vi "Format CSV.vi"(8 "error in (no error)":errorcluster, 9 "delimiter":string=",", 10 "CSV File Input":path, 11 "Original CSV Format":enum16{"Format A", "Format B"}(ring)) -> (0 "error out":errorcluster, 1 "Parcel Length":i32[](array[numeric]), 2 "All Terminal Data":T1(array[cluster]))   [LabVIEW 2017] (continued)
"38:45.8", "38:45.9", "38:45.9", "38:45.9", "38:46.0", "38:46.0", "38:46.0", "38:46.1", "38:46.1", "38:46.1", "38:46.2", "38:46.2", "38:46.2", "38:46.3", "38:46.3", "38:46.3", "38:46.4", "38:46.4", "38:46.4", "38:46.5", "38:46.5", "38:46.5", "38:46.6", "38:46.6", "38:46.6", "38:46.7", "38:46.7", "38:46.7", "38:46.8", "38:46.8", "38:46.8", "38:46.9", "38:46.9", "38:46.9", "38:47.0", "38:47.0", "38:47.0", "38:47.1", "38:47.1", "38:47.1", "38:47.2", "38:47.2", "38:47.2", "38:47.3", "38:47.3", "38:47.3", "38:47.4", "38:47.4", "38:47.4", "38:47.5", "38:47.5", "38:47.5", "38:47.6", "38:47.6", "38:47.6", "38:47.7", "38:47.7", "38:47.7", "38:47.8", "38:47.8", "38:47.8", "38:47.9", "38:47.9", "38:47.9", "38:48.0", "38:48.0", "38:48.0", "38:48.1", "38:48.1", "38:48.1", "38:48.2", "38:48.2", "38:48.2", "38:48.3", "38:48.3", "38:48.3", "38:48.4", "38:48.4", "38:48.4", "38:48.5", "38:48.5", "38:48.5", "38:48.6", "38:48.6", "38:48.6", "38:48.7", "38:48.7", "38:48.7", "38:48.8", "38:48.8", "38:48.8", "38:48.9", "38:48.9", "38:48.9", "38:49.0", "38:49.0", "38:49.0", "38:49.1", "38:49.1", "38:49.1", "38:49.2", "38:49.2", "38:49.2", "38:49.3", "38:49.3", "38:49.3", "38:49.4", "38:49.4", "38:49.4", "38:49.5", "38:49.5", "38:49.5", "38:49.6", "38:49.6", "38:49.6", "38:49.7", "38:49.7", "38:49.7", "38:49.8", "38:49.8", "38:49.8", "38:49.9", "38:49.9", "38:49.9", "38:50.0", "38:50.0", "38:50.0", "38:50.1", "38:50.1", "38:50.1", "38:50.2", "38:50.2", "38:50.2", "38:50.3", "38:50.3", "38:50.3", "38:50.4", "38:50.4", "38:50.4", "38:50.5", "38:50.5", "38:50.5", "38:50.6", "38:50.6", "38:50.6", "38:50.7", "38:50.7", "38:50.7", "38:50.8", "38:50.8", "38:50.8", "38:50.9", "38:50.9", "38:50.9", "38:51.0", "38:51.0", "38:51.0", "38:51.1", "38:51.1", "38:51.1", "38:51.2", "38:51.2", "38:51.2", "38:51.3", "38:51.3", "38:51.3", "38:51.4", "38:51.4", "38:51.4", "38:51.5", "38:51.5", "38:51.5", "38:51.6", "38:51.6", "38:51.6", "38:51.7", "38:51.7", "38:51.7", "38:51.8", "38:51.8", "38:51.8", "38:51.9", "38:51.9", "38:51.9", "38:52.0", "38:52.0", "38:52.0", "38:52.1", "38:52.1", "38:52.1", "38:52.2", "38:52.2", "38:52.2", "38:52.3", "38:52.3", "38:52.3", "38:52.4", "38:52.4", "38:52.4", "38:52.5", "38:52.5", "38:52.5", "38:52.6", "38:52.6", "38:52.6", "38:52.7", "38:52.7", "38:52.7", "38:52.8", "38:52.8", "38:52.8", "38:52.9", "38:52.9", "38:52.9", "38:53.0", "38:53.0", "38:53.0", "38:53.1", "38:53.1", "38:53.1", "38:53.2", "38:53.2", "38:53.2", "38:53.3", "38:53.3", "38:53.3", "38:53.4", "38:53.4", "38:53.4", "38:53.5", "38:53.5", "38:53.5", "38:53.6", "38:53.6", "38:53.6", "38:53.7", "38:53.7", "38:53.7", "38:53.8", "38:53.8", "38:53.8", "38:53.9", "38:53.9", "38:53.9", "38:54.0", "38:54.0", "38:54.0", "38:54.1", "38:54.1", "38:54.1", "38:54.2", "38:54.2", "38:54.2", "38:54.3", "38:54.3", "38:54.3", "38:54.4", "38:54.4", "38:54.4", "38:54.5", "38:54.5", "38:54.5", "38:54.6", "38:54.6", "38:54.6", "38:54.7", "38:54.7", "38:54.7", "38:54.8", "38:54.8", "38:54.8", "38:54.9", "38:54.9", "38:54.9", "38:55.0", "38:55.0", "38:55.0", "38:55.1", "38:55.1", "38:55.1", "38:55.2", "38:55.2", "38:55.2", "38:55.3", "38:55.3", "38:55.3", "38:55.4", "38:55.4", "38:55.4", "38:55.5", "38:55.5", "38:55.5", "38:55.6", "38:55.6", "38:55.6", "38:55.7", "38:55.7", "38:55.7", "38:55.8", "38:55.8", "38:55.8", "38:55.9", "38:55.9", "38:55.9", "38:56.0", "38:56.0", "38:56.0", "38:56.1", "38:56.1", "38:56.1", "38:56.2", "38:56.2", "38:56.2", "38:56.3", "38:56.3", "38:56.3", "38:56.4", "38:56.4", "38:56.4", "38:56.5", "38:56.5", "38:56.5", "38:56.6", "38:56.6", "38:56.6", "38:56.7", "38:56.7", "38:56.7", "38:56.8", "38:56.8", "38:56.8", "38:56.9", "38:56.9", "38:56.9", "38:57.0", "38:57.0", "38:57.0", "38:57.1", "38:57.1", "38:57.1", "38:57.2", "38:57.2", "38:57.2", "38:57.3", "38:57.3", "38:57.3", "38:57.4", "38:57.4", "38:57.4", "38:57.5", "38:57.5", "38:57.5", "38:57.6", "38:57.6", "38:57.6", "38:57.7", "38:57.7", "38:57.7", "38:57.8", "38:57.8", "38:57.8", "38:57.9", "38:57.9", "38:57.9", "38:58.0", "38:58.0", "38:58.0", "38:58.1", "38:58.1", "38:58.1", "38:58.2", "38:58.2", "38:58.2", "38:58.3", "38:58.3", "38:58.3", "38:58.4", "38:58.4", "38:58.4", "38:58.5", "38:58.5", "38:58.5", "38:58.6", "38:58.6", "38:58.6", "38:58.7", "38:58.7", "38:58.7", "38:58.8", "38:58.8", "38:58.8", "38:58.9", "38:58.9", "38:58.9", "38:59.0", "38:59.0", "38:59.0", "38:59.1", "38:59.1", "38:59.1", "38:59.2", "38:59.2", "38:59.2", "38:59.3", "38:59.3", "38:59.3", "38:59.4", "38:59.4", "38:59.4", "38:59.5", "38:59.5", "38:59.5", "38:59.6", "38:59.6", "38:59.6", "38:59.7", "38:59.7", "38:59.7", "38:59.8", "38:59.8", "38:59.8", "38:59.9", "38:59.9", "38:59.9", "39:00.0", "39:00.0", "39:00.0", "39:00.1", "39:00.1", "39:00.1", "39:00.2", "39:00.2", "39:00.2", "39:00.3", "39:00.3", "39:00.3", "39:00.4", "39:00.4", "39:00.4", "39:00.5", "39:00.5", "39:00.5", "39:00.6", "39:00.6", "39:00.6", "39:00.7", "39:00.7", "39:00.7", "39:00.8", "39:00.8", "39:00.8", "39:00.9", "39:00.9", "39:00.9", "39:01.0", "39:01.0", "39:01.0", "39:01.1", "39:01.1", "39:01.1", "39:01.2", "39:01.2", "39:01.2", "39:01.3", "39:01.3", "39:01.3", "39:01.4", "39:01.4", "39:01.4", "39:01.5", "39:01.5", "39:01.5", "39:01.6", "39:01.6", "39:01.6", "39:01.7", "39:01.7", "39:01.7", "39:01.8", "39:01.8", "39:01.8", "39:01.9", "39:01.9", "39:01.9", "39:02.0", "39:02.0", "39:02.0", "39:02.1", "39:02.1", "39:02.1", "39:02.2", "39:02.2", "39:02.2", "39:02.3", "39:02.3", "39:02.3", "39:02.4", "39:02.4", "39:02.4", "39:02.5", "39:02.5", "39:02.5", "39:02.6", "39:02.6", "39:02.6", "39:02.7", "39:02.7", "39:02.7", "39:02.8", "39:02.8", "39:02.8", "39:02.9", "39:02.9", "39:02.9", "39:03.0", "39:03.0", "39:03.0", "39:03.1", "39:03.1", "39:03.1", "39:03.2", "39:03.2", "39:03.2", "39:03.3", "39:03.3", "39:03.3", "39:03.4", "39:03.4", "39:03.4", "39:03.5", "39:03.5", "39:03.5", "39:03.6", "39:03.6", "39:03.6", "39:03.7", "39:03.7", "39:03.7", "39:03.8", "39:03.8", "39:03.8", "39:03.9", "39:03.9", "39:03.9", "39:04.0", "39:04.0", "39:04.0", "39:04.1", "39:04.1", "39:04.1", "39:04.2", "39:04.2", "39:04.2", "39:04.3", "39:04.3", "39:04.3", "39:04.4", "39:04.4", "39:04.4", "39:04.5", "39:04.5", "39:04.5", "39:04.6", "39:04.6", "39:04.6", "39:04.7", "39:04.7", "39:04.7", "39:04.8", "39:04.8", "39:04.8", "39:04.9", "39:04.9", "39:04.9", "39:05.0", "39:05.0", "39:05.0", "39:05.1", "39:05.1", "39:05.1", "39:05.2", "39:05.2", "39:05.2", "39:05.3", "39:05.3", "39:05.3", "39:05.4", "39:05.4", "39:05.4", "39:05.5", "39:05.5", "39:05.5", "39:05.6", "39:05.6", "39:05.6", "39:05.7", "39:05.7", "39:05.7", "39:05.8", "39:05.8", "39:05.8", "39:05.9", "39:05.9", "39:05.9", "39:06.0", "39:06.0", "39:06.0", "39:06.1", "39:06.1", "39:06.1", "39:06.2", "39:06.2", "39:06.2", "39:06.3", "39:06.3", "39:06.3", "39:06.4", "39:06.4", "39:06.4", "39:06.5", "39:06.5", "39:06.5", "39:06.6", "39:06.6", "39:06.6", "39:06.7", "39:06.7", "39:06.7", "39:06.8", "39:06.8", "39:06.8", "39:06.9", "39:06.9", "39:06.9", "39:07.0", "39:07.0", "39:07.0", "39:07.1", "39:07.1", "39:07.1", "39:07.2", "39:07.2", "39:07.2", "39:07.3", "39:07.3", "39:07.3", "39:07.4", "39:07.4", "39:07.4", "39:07.5", "39:07.5", "39:07.5", "39:07.6", "39:07.6", "39:07.6", "39:07.7", "39:07.7", "39:07.7", "39:07.8", "39:07.8", "39:07.8", "39:07.9", "39:07.9", "39:07.9", "39:08.0", "39:08.0", "39:08.0", "39:08.1", "39:08.1", "39:08.1", "39:08.2", "39:08.2", "39:08.2", "39:08.3", "39:08.3", "39:08.3", "39:08.4", "39:08.4", "39:08.4", "39:08.5", "39:08.5", "39:08.5", "39:08.6", "39:08.6", "39:08.6", "39:08.7", "39:08.7", "39:08.7", "39:08.8", "39:08.8", "39:08.8", "39:08.9", "39:08.9", "39:08.9", "39:09.0", "39:09.0", "39:09.0", "39:09.1", "39:09.1", "39:09.1", "39:09.2", "39:09.2", "39:09.2", "39:09.3", "39:09.3", "39:09.3", "39:09.4", "39:09.4", "39:09.4", "39:09.5", "39:09.5", "39:09.5", "39:09.6", "39:09.6", "39:09.6", "39:09.7", "39:09.7", "39:09.7", "39:09.8", "39:09.8", "39:09.8", "39:09.9", "39:09.9", "39:09.9", "39:10.0", "39:10.0", "39:10.0", "39:10.1", "39:10.1", "39:10.1", "39:10.2", "39:10.2", "39:10.2", "39:10.3", "39:10.3", "39:10.3", "39:10.4", "39:10.4", "39:10.4", "39:10.5", "39:10.5", "39:10.5", "39:10.6", "39:10.6", "39:10.6", "39:10.7", "39:10.7", "39:10.7", "39:10.8", "39:10.8", "39:10.8", "39:10.9", "39:10.9", "39:10.9", "39:11.0", "39:11.0", "39:11.0", "39:11.1", "39:11.1", "39:11.1", "39:11.2", "39:11.2", "39:11.2", "39:11.3", "39:11.3", "39:11.3", "39:11.4", "39:11.4", "39:11.4", "39:11.5", "39:11.5", "39:11.5", "39:11.6", "39:11.6", "39:11.6", "39:11.7", "39:11.7", "39:11.7", "39:11.8", "39:11.8", "39:11.8", "39:11.9", "39:11.9", "39:11.9", "39:12.0", "39:12.0", "39:12.0", "39:12.1", "39:12.1", "39:12.1", "39:12.2", "39:12.2", "39:12.2", "39:12.3", "39:12.3", "39:12.3", "39:12.4", "39:12.4", "39:12.4", "39:12.5", "39:12.5", "39:12.5", "39:12.6", "39:12.6", "39:12.6", "39:12.7", "39:12.7", "39:12.7", "39:12.8", "39:12.8", "39:12.8", "39:12.9", "39:12.9", "39:12.9", "39:13.0", "39:13.0", "39:13.0", "39:13.1", "39:13.1", "39:13.1", "39:13.2", "39:13.2", "39:13.2", "39:13.3", "39:13.3", "39:13.3", "39:13.4", "39:13.4", "39:13.4", "39:13.5", "39:13.5", "39:13.5", "39:13.6", "39:13.6", "39:13.6", "39:13.7", "39:13.7", "39:13.7", "39:13.8", "39:13.8", "39:13.8", "39:13.9", "39:13.9", "39:13.9", "39:14.0", "39:14.0", "39:14.0", "39:14.1", "39:14.1", "39:14.1", "39:14.2", "39:14.2", "39:14.2", "39:14.3", "39:14.3", "39:14.3", "39:14.4", "39:14.4", "39:14.4", "39:14.5", "39:14.5", "39:14.5", "39:14.6", "39:14.6", "39:14.6", "39:14.7", "39:14.7", "39:14.7", "39:14.8", "39:14.8", "39:14.8", "39:14.9", "39:14.9", "39:14.9", "39:15.0", "39:15.0", "39:15.0", "39:15.1", "39:15.1", "39:15.1", "39:15.2", "39:15.2", "39:15.2", "39:15.3", "39:15.3", "39:15.3", "39:15.4", "39:15.4", "39:15.4", "39:15.5", "39:15.5", "39:15.5", "39:15.6", "39:15.6", "39:15.6", "39:15.7", "39:15.7", "39:15.7", "39:15.8", "39:15.8", "39:15.8", "39:15.9", "39:15.9", "39:15.9", "39:16.0", "39:16.0", "39:16.0", "39:16.1", "39:16.1", "39:16.1", "39:16.2", "39:16.2", "39:16.2", "39:16.3", "39:16.3", "39:16.3", "39:16.4", "39:16.4", "39:16.4", "39:16.5", "39:16.5", "39:16.5", "39:16.6", "39:16.6", "39:16.6", "39:16.7", "39:16.7", "39:16.7", "39:16.8", "39:16.8", "39:16.8", "39:16.9", "39:16.9", "39:16.9", "39:17.0", "39:17.0", "39:17.0", "39:17.1", "39:17.1", "39:17.1", "39:17.2", "39:17.2", "39:17.2", "39:17.3", "39:17.3", "39:17.3", "39:17.4", "39:17.4", "39:17.4", "39:17.5", "39:17.5", "39:17.5", "39:17.6", "39:17.6", "39:17.6", "39:17.7", "39:17.7", "39:17.7", "39:17.8", "39:17.8", "39:17.8", "39:17.9", "39:17.9", "39:17.9", "39:18.0", "39:18.0", "39:18.0", "39:18.1", "39:18.1", "39:18.1", "39:18.2", "39:18.2", "39:18.2", "39:18.3", "39:18.3", "39:18.3", "39:18.4", "39:18.4", "39:18.4", "39:18.5", "39:18.5", "39:18.5", "39:18.6", "39:18.6", "39:18.6", "39:18.7", "39:18.7", "39:18.7", "39:18.8", "39:18.8", "39:18.8", "39:18.9", "39:18.9", "39:18.9", "39:19.0", "39:19.0", "39:19.0", "39:19.1", "39:19.1", "39:19.1", "39:19.2", "39:19.2", "39:19.2", "39:19.3", "39:19.3", "39:19.3", "39:19.4", "39:19.4", "39:19.4", "39:19.5", "39:19.5", "39:19.5", "39:19.6", "39:19.6", "39:19.6", "39:19.7", "39:19.7", "39:19.7", "39:19.8", "39:19.8", "39:19.8", "39:19.9", "39:19.9", "39:19.9", "39:20.0", "39:20.0", "39:20.0", "39:20.1", "39:20.1", "39:20.1", "39:20.2", "39:20.2", "39:20.2", "39:20.3", "39:20.3", "39:20.3", "39:20.4", "39:20.4", "39:20.4", "39:20.5", "39:20.5", "39:20.5", "39:20.6", "39:20.6", "39:20.6", "39:20.7", "39:20.7", "39:20.7", "39:20.8", "39:20.8", "39:20.8", "39:20.9", "39:20.9", "39:20.9", "39:21.0", "39:21.0", "39:21.0", "39:21.1", "39:21.1", "39:21.1", "39:21.2", "39:21.2", "39:21.2", "39:21.3", "39:21.3", "39:21.3", "39:21.4", "39:21.4", "39:21.4", "39:21.5", "39:21.5", "39:21.5", "39:21.6", "39:21.6", "39:21.6", "39:21.7", "39:21.7", "39:21.7", "39:21.8", "39:21.8", "39:21.8", "39:21.9", "39:21.9", "39:21.9", "39:22.0", "39:22.0", "39:22.0", "39:22.1", "39:22.1", "39:22.1", "39:22.2", "39:22.2", "39:22.2", "39:22.3", "39:22.3", "39:22.3", "39:22.4", "39:22.4", "39:22.4", "39:22.5", "39:22.5", "39:22.5", "39:22.6", "39:22.6", "39:22.6", "39:22.7", "39:22.7", "39:22.7", "39:22.8", "39:22.8", "39:22.8", "39:22.9", "39:22.9", "39:22.9", "39:23.0", "39:23.0", "39:23.0", "39:23.1", "39:23.1", "39:23.1", "39:23.2", "39:23.2", "39:23.2", "39:23.3", "39:23.3", "39:23.3", "39:23.4", "39:23.4", "39:23.4", "39:23.5", "39:23.5", "39:23.5", "39:23.6", "39:23.6", "39:23.6", "39:23.7", "39:23.7", "39:23.7", "39:23.8", "39:23.8", "39:23.8", "39:23.9", "39:23.9", "39:23.9", "39:24.0", "39:24.0", "39:24.0", "39:24.1", "39:24.1", "39:24.1", "39:24.2", "39:24.2", "39:24.2", "39:24.3", "39:24.3", "39:24.3", "39:24.4", "39:24.4", "39:24.4", "39:24.5", "39:24.5", "39:24.5", "39:24.6", "39:24.6", "39:24.6", "39:24.7", "39:24.7", "39:24.7", "39:24.8", "39:24.8", "39:24.8", "39:24.9", "39:24.9", "39:24.9", "39:25.0", "39:25.0", "39:25.0", "39:25.1", "39:25.1", "39:25.1", "39:25.2", "39:25.2", "39:25.2", "39:25.3", "39:25.3", "39:25.3", "39:25.4", "39:25.4", "39:25.4", "39:25.5", "39:25.5", "39:25.5", "39:25.6", "39:25.6", "39:25.6", "39:25.7", "39:25.7", "39:25.7", "39:25.8", "39:25.8", "39:25.8", "39:25.9", "39:25.9", "39:25.9", "39:26.0", "39:26.0", "39:26.0", "39:26.1", "39:26.1", "39:26.1", "39:26.2", "39:26.2", "39:26.2", "39:26.3", "39:26.3", "39:26.3", "39:26.4", "39:26.4", "39:26.4", "39:26.5", "39:26.5", "39:26.5", "39:26.6", "39:26.6", "39:26.6", "39:26.7", "39:26.7", "39:26.7", "39:26.8", "39:26.8", "39:26.8", "39:26.9", "39:26.9", "39:26.9", "39:27.0", "39:27.0", "39:27.0", "39:27.1", "39:27.1", "39:27.1", "39:27.2", "39:27.2", "39:27.2", "39:27.3", "39:27.3", "39:27.3", "39:27.4", "39:27.4", "39:27.4", "39:27.5", "39:27.5", "39:27.5", "39:27.6", "39:27.6", "39:27.6", "39:27.7", "39:27.7", "39:27.7", "39:27.8", "39:27.8", "39:27.8", "39:27.9", "39:27.9", "39:27.9", "39:28.0", "39:28.0", "39:28.0", "39:28.1", "39:28.1", "39:28.1", "39:28.2", "39:28.2", "39:28.2", "39:28.3", "39:28.3", "39:28.3", "39:28.4", "39:28.4", "39:28.4", "39:28.5", "39:28.5", "39:28.5", "39:28.6", "39:28.6", "39:28.6", "39:28.7", "39:28.7", "39:28.7", "39:28.8", "39:28.8", "39:28.8", "39:28.9", "39:28.9", "39:28.9", "39:29.0", "39:29.0", "39:29.0", "39:29.1", "39:29.1", "39:29.1", "39:29.2", "39:29.2", "39:29.2", "39:29.3", "39:29.3", "39:29.3", "39:29.4", "39:29.4", "39:29.4", "39:29.5", "39:29.5", "39:29.5", "39:29.6", "39:29.6", "39:29.6", "39:29.7", "39:29.7", "39:29.7", "39:29.8", "39:29.8", "39:29.8", "39:29.9", "39:29.9", "39:29.9", "39:30.0", "39:30.0", "39:30.0", "39:30.1", "39:30.1", "39:30.1", "39:30.2", "39:30.2", "39:30.2", "39:30.3", "39:30.3", "39:30.3", "39:30.4", "39:30.4", "39:30.4", "39:30.5", "39:30.5", "39:30.5", "39:30.6", "39:30.6", "39:30.6", "39:30.7", "39:30.7", "39:30.7", "39:30.8", "39:30.8", "39:30.8", "39:30.9", "39:30.9", "39:30.9", "39:31.0", "39:31.0", "39:31.0", "39:31.1", "39:31.1", "39:31.1", "39:31.2", "39:31.2", "39:31.2", "39:31.3", "39:31.3", "39:31.3", "39:31.4", "39:31.4", "39:31.4", "39:31.5", "39:31.5", "39:31.5", "39:31.6", "39:31.6", "39:31.6", "39:31.7", "39:31.7", "39:31.7", "39:31.8", "39:31.8", "39:31.8", "39:31.9", "39:31.9", "39:31.9", "39:32.0", "39:32.0", "39:32.0", "39:32.1", "39:32.1", "39:32.1", "39:32.2", "39:32.2", "39:32.2", "39:32.3", "39:32.3", "39:32.3", "39:32.4", "39:32.4", "39:32.4", "39:32.5", "39:32.5", "39:32.5", "39:32.6", "39:32.6", "39:32.6", "39:32.7", "39:32.7", "39:32.7", "39:32.8", "39:32.8", "39:32.8", "39:32.9", "39:32.9", "39:32.9", "39:33.0", "39:33.0", "39:33.0", "39:33.1", "39:33.1", "39:33.1", "39:33.2", "39:33.2", "39:33.2", "39:33.3", "39:33.3", "39:33.3", "39:33.4", "39:33.4", "39:33.4", "39:33.5", "39:33.5", "39:33.5", "39:33.6", "39:33.6", "39:33.6", "39:33.7", "39:33.7", "39:33.7", "39:33.8", "39:33.8", "39:33.8", "39:33.9", "39:33.9", "39:33.9", "39:34.0", "39:34.0", "39:34.0", "39:34.1", "39:34.1", "39:34.1", "39:34.2", "39:34.2", "39:34.2", "39:34.3", "39:34.3", "39:34.3", "39:34.4", "39:34.4", "39:34.4", "39:34.5", "39:34.5", "39:34.5", "39:34.6", "39:34.6", "39:34.6", "39:34.7", "39:34.7", "39:34.7", "39:34.8", "39:34.8", "39:34.8", "39:34.9", "39:34.9", "39:34.9", "39:35.0", "39:35.0", "39:35.0", "39:35.1", "39:35.1", "39:35.1", "39:35.2", "39:35.2", "39:35.2", "39:35.3", "39:35.3", "39:35.3", "39:35.4", "39:35.4", "39:35.4", "39:35.5", "39:35.5", "39:35.5", "39:35.6", "39:35.6", "39:35.6", "39:35.7", "39:35.7", "39:35.7", "39:35.8", "39:35.8", "39:35.8", "39:35.9", "39:35.9", "39:35.9", "39:36.0", "39:36.0", "39:36.0", "39:36.1", "39:36.1", "39:36.1", "39:36.2", "39:36.2", "39:36.2", "39:36.3", "39:36.3", "39:36.3", "39:36.4", "39:36.4", "39:36.4", "39:36.5", "39:36.5", "39:36.5", "39:36.6", "39:36.6", "39:36.6", "39:36.7", "39:36.7", "39:36.7", "39:36.8", "39:36.8", "39:36.8", "39:36.9", "39:36.9", "39:36.9", "39:37.0", "39:37.0", "39:37.0", "39:37.1", "39:37.1", "39:37.1", "39:37.2", "39:37.2", "39:37.2", "39:37.3", "39:37.3", "39:37.3", "39:37.4", "39:37.4", "39:37.4", "39:37.5", "39:37.5", "39:37.5", "39:37.6", "39:37.6", "39:37.6", "39:37.7", "39:37.7", "39:37.7", "39:37.8", "39:37.8", "39:37.8", "39:37.9", "39:37.9", "39:37.9", "39:38.0", "39:38.0", "39:38.0", "39:38.1", "39:38.1", "39:38.1", "39:38.2", "39:38.2", "39:38.2", "39:38.3", "39:38.3", "39:38.3", "39:38.4", "39:38.4", "39:38.4", "39:38.5", "39:38.5", "39:38.5", "39:38.6", "39:38.6", "39:38.6", "39:38.7", "39:38.7", "39:38.7", "39:38.8", "39:38.8", "39:38.8", "39:38.9", "39:38.9", "39:38.9", "39:39.0", "39:39.0", "39:39.0", "39:39.1", "39:39.1", "39:39.1", "39:39.2", "39:39.2", "39:39.2", "39:39.3", "39:39.3", "39:39.3", "39:39.4", "39:39.4", "39:39.4", "39:39.5", "39:39.5", "39:39.5", "39:39.6", "39:39.6", "39:39.6", "39:39.7", "39:39.7", "39:39.7", "39:39.8", "39:39.8", "39:39.8", "39:39.9", "39:39.9", "39:39.9", "39:40.0", "39:40.0", "39:40.0", "39:40.1", "39:40.1", "39:40.1", "39:40.2", "39:40.2", "39:40.2", "39:40.3", "39:40.3", "39:40.3", "39:40.4", "39:40.4", "39:40.4", "39:40.5", "39:40.5", "39:40.5", "39:40.6", "39:40.6", "39:40.6", "39:40.7", "39:40.7", "39:40.7", "39:40.8", "39:40.8", "39:40.8", "39:40.9", "39:40.9", "39:40.9", "39:41.0", "39:41.0", "39:41.0", "39:41.1", "39:41.1", "39:41.1", "39:41.2", "39:41.2", "39:41.2", "39:41.3", "39:41.3", "39:41.3", "39:41.4", "39:41.4", "39:41.4", "39:41.5", "39:41.5", "39:41.5", "39:41.6", "39:41.6", "39:41.6", "39:41.7", "39:41.7", "39:41.7", "39:41.8", "39:41.8", "39:41.8", "39:41.9", "39:41.9", "39:41.9", "39:42.0", "39:42.0", "39:42.0", "39:42.1", "39:42.1", "39:42.1", "39:42.2", "39:42.2", "39:42.2", "39:42.3", "39:42.3", "39:42.3", "39:42.4", "39:42.4", "39:42.4", "39:42.5", "39:42.5", "39:42.5", "39:42.6", "39:42.6", "39:42.6", "39:42.7", "39:42.7", "39:42.7", "39:42.8", "39:42.8", "39:42.8", "39:42.9", "39:42.9", "39:42.9", "39:43.0", "39:43.0", "39:43.0", "39:43.1", "39:43.1", "39:43.1", "39:43.2", "39:43.2", "39:43.2", "39:43.3", "39:43.3", "39:43.3", "39:43.4", "39:43.4", "39:43.4", "39:43.5", "39:43.5", "39:43.5", "39:43.6", "39:43.6", "39:43.6", "39:43.7", "39:43.7", "39:43.7", "39:43.8", "39:43.8", "39:43.8", "39:43.9", "39:43.9", "39:43.9", "39:44.0", "39:44.0", "39:44.0", "39:44.1", "39:44.1", "39:44.1", "39:44.2", "39:44.2", "39:44.2", "39:44.3", "39:44.3", "39:44.3", "39:44.4", "39:44.4", "39:44.4", "39:44.5", "39:44.5", "39:44.5", "39:44.6", "39:44.6", "39:44.6", "39:44.7", "39:44.7", "39:44.7", "39:44.8", "39:44.8", "39:44.8", "39:44.9", "39:44.9", "39:44.9", "39:45.0", "39:45.0", "39:45.0", "39:45.1", "39:45.1", "39:45.1", "39:45.2", "39:45.2", "39:45.2", "39:45.3", "39:45.3", "39:45.3", "39:45.4", "39:45.4", "39:45.4", "39:45.5", "39:45.5", "39:45.5", "39:45.6", "39:45.6", "39:45.6", "39:45.7", "39:45.7", "39:45.7", "39:45.8", "39:45.8", "39:45.8", "39:45.9", "39:45.9", "39:45.9", "39:46.0", "39:46.0", "39:46.0", "39:46.1", "39:46.1", "39:46.1", "39:46.2", "39:46.2", "39:46.2", "39:46.3", "39:46.3", "39:46.3", "39:46.4", "39:46.4", "39:46.4", "39:46.5", "39:46.5", "39:46.5", "39:46.6", "39:46.6", "39:46.6", "39:46.7", "39:46.7", "39:46.7", "39:46.8", "39:46.8", "39:46.8", "39:46.9", "39:46.9", "39:46.9", "39:47.0", "39:47.0", "39:47.0", "39:47.1", "39:47.1", "39:47.1", "39:47.2", "39:47.2", "39:47.2", "39:47.3", "39:47.3", "39:47.3", "39:47.4", "39:47.4", "39:47.4", "39:47.5", "39:47.5", "39:47.5", "39:47.6", "39:47.6", "39:47.6", "39:47.7", "39:47.7", "39:47.7", "39:47.8", "39:47.8", "39:47.8", "39:47.9", "39:47.9", "39:47.9", "39:48.0", "39:48.0", "39:48.0", "39:48.1", "39:48.1", "39:48.1", "39:48.2", "39:48.2", "39:48.2", "39:48.3", "39:48.3", "39:48.3", "39:48.4", "39:48.4", "39:48.4", "39:48.5", "39:48.5", "39:48.5", "39:48.6", "39:48.6", "39:48.6", "39:48.7", "39:48.7", "39:48.7", "39:48.8", "39:48.8", "39:48.8", "39:48.9", "39:48.9", "39:48.9", "39:49.0", "39:49.0", "39:49.0", "39:49.1", "39:49.1", "39:49.1", "39:49.2", "39:49.2", "39:49.2", "39:49.3", "39:49.3", "39:49.3", "39:49.4", "39:49.4", "39:49.4", "39:49.5", "39:49.5", "39:49.5", "39:49.6", "39:49.6", "39:49.6", "39:49.7", "39:49.7", "39:49.7", "39:49.8", "39:49.8", "39:49.8", "39:49.9", "39:49.9", "39:49.9", "39:50.0", "39:50.0", "39:50.0", "39:50.1", "39:50.1", "39:50.1", "39:50.2", "39:50.2", "39:50.2", "39:50.3", "39:50.3", "39:50.3", "39:50.4", "39:50.4", "39:50.4", "39:50.5", "39:50.5", "39:50.5", "39:50.6", "39:50.6", "39:50.6", "39:50.7", "39:50.7", "39:50.7", "39:50.8", "39:50.8", "39:50.8", "39:50.9", "39:50.9", "39:50.9", "39:51.0", "39:51.0", "39:51.0", "39:51.1", "39:51.1", "39:51.1", "39:51.2", "39:51.2", "39:51.2", "39:51.3", "39:51.3", "39:51.3", "39:51.4", "39:51.4", "39:51.4", "39:51.5", "39:51.5", "39:51.5", "39:51.6", "39:51.6", "39:51.6", "39:51.7", "39:51.7", "39:51.7", "39:51.8", "39:51.8", "39:51.8", "39:51.9", "39:51.9", "39:51.9", "39:52.0", "39:52.0", "39:52.0", "39:52.1", "39:52.1", "39:52.1", "39:52.2", "39:52.2", "39:52.2", "39:52.3", "39:52.3", "39:52.3", "39:52.4", "39:52.4", "39:52.4", "39:52.5", "39:52.5", "39:52.5", "39:52.6", "39:52.6", "39:52.6", "39:52.7", "39:52.7", "39:52.7", "39:52.8", "39:52.8", "39:52.8", "39:52.9", "39:52.9", "39:52.9", "39:53.0", "39:53.0", "39:53.0", "39:53.1", "39:53.1", "39:53.1", "39:53.2", "39:53.2", "39:53.2", "39:53.3", "39:53.3", "39:53.3", "39:53.4", "39:53.4", "39:53.4", "39:53.5", "39:53.5", "39:53.5", "39:53.6", "39:53.6", "39:53.6", "39:53.7", "39:53.7", "39:53.7", "39:53.8", "39:53.8", "39:53.8", "39:53.9", "39:53.9", "39:53.9", "39:54.0", "39:54.0", "39:54.0", "39:54.1", "39:54.1", "39:54.1", "39:54.2", "39:54.2", "39:54.2", "39:54.3", "39:54.3", "39:54.3", "39:54.4", "39:54.4", "39:54.4", "39:54.5", "39:54.5", "39:54.5", "39:54.6", "39:54.6", "39:54.6", "39:54.7", "39:54.7", "39:54.7", "39:54.8", "39:54.8", "39:54.8", "39:54.9", "39:54.9", "39:54.9", "39:55.0", "39:55.0", "39:55.0", "39:55.1", "39:55.1", "39:55.1", "39:55.2", "39:55.2", "39:55.2", "39:55.3", "39:55.3", "39:55.3", "39:55.4", "39:55.4", "39:55.4", "39:55.5", "39:55.5", "39:55.5", "39:55.6", "39:55.6", "39:55.6", "39:55.7", "39:55.7", "39:55.7", "39:55.8", "39:55.8", "39:55.8", "39:55.9", "39:55.9", "39:55.9", "39:56.0", "39:56.0", "39:56.0", "39:56.1", "39:56.1", "39:56.1", "39:56.2", "39:56.2", "39:56.2", "39:56.3", "39:56.3", "39:56.3", "39:56.4", "39:56.4", "39:56.4", "39:56.5", "39:56.5", "39:56.5", "39:56.6", "39:56.6", "39:56.6", "39:56.7", "39:56.7", "39:56.7", "39:56.8", "39:56.8", "39:56.8", "39:56.9", "39:56.9", "39:56.9", "39:57.0", "39:57.0", "39:57.0", "39:57.1", "39:57.1", "39:57.1", "39:57.2", "39:57.2", "39:57.2", "39:57.3", "39:57.3", "39:57.3", "39:57.4", "39:57.4", "39:57.4", "39:57.5", "39:57.5", "39:57.5", "39:57.6", "39:57.6", "39:57.6", "39:57.7", "39:57.7", "39:57.7", "39:57.8", "39:57.8", "39:57.8", "39:57.9", "39:57.9", "39:57.9", "39:58.0", "39:58.0", "39:58.0", "39:58.1", "39:58.1", "39:58.1", "39:58.2", "39:58.2", "39:58.2", "39:58.3", "39:58.3", "39:58.3", "39:58.4", "39:58.4", "39:58.4", "39:58.5", "39:58.5", "39:58.5", "39:58.6", "39:58.6", "39:58.6", "39:58.7", "39:58.7", "39:58.7", "39:58.8", "39:58.8", "39:58.8", "39:58.9", "39:58.9", "39:58.9", "39:59.0", "39:59.0", "39:59.0", "39:59.1", "39:59.1", "39:59.1", "39:59.2", "39:59.2", "39:59.2", "39:59.3", "39:59.3", "39:59.3", "39:59.4", "39:59.4", "39:59.4", "39:59.5", "39:59.5", "39:59.5", "39:59.6", "39:59.6", "39:59.6", "39:59.7", "39:59.7", "39:59.7", "39:59.8", "39:59.8", "39:59.8", "39:59.9", "39:59.9", "39:59.9", "40:00.0", "40:00.0", "40:00.0", "40:00.1", "40:00.1", "40:00.1", "40:00.2", "40:00.2", "40:00.2", "40:00.3", "40:00.3", "40:00.3", "40:00.4", "40:00.4", "40:00.4", "40:00.5", "40:00.5", "40:00.5", "40:00.6", "40:00.6", "40:00.6", "40:00.7", "40:00.7", "40:00.7", "40:00.8", "40:00.8", "40:00.8", "40:00.9", "40:00.9", "40:00.9", "40:01.0", "40:01.0", "40:01.0", "40:01.1", "40:01.1", "40:01.1", "40:01.2", "40:01.2", "40:01.2", "40:01.3", "40:01.3", "40:01.3", "40:01.4", "40:01.4", "40:01.4", "40:01.5", "40:01.5", "40:01.5", "40:01.6", "40:01.6", "40:01.6", "40:01.7", "40:01.7", "40:01.7", "40:01.8", "40:01.8", "40:01.8", "40:01.9", "40:01.9", "40:01.9", "40:02.0", "40:02.0", "40:02.0", "40:02.1", "40:02.1", "40:02.1", "40:02.2", "40:02.2", "40:02.2", "40:02.3", "40:02.3", "40:02.3", "40:02.4", "40:02.4", "40:02.4", "40:02.5", "40:02.5", "40:02.5", "40:02.6", "40:02.6", "40:02.6", "40:02.7", "40:02.7", "40:02.7", "40:02.8", "40:02.8", "40:02.8", "40:02.9", "40:02.9", "40:02.9", "40:03.0", "40:03.0", "40:03.0", "40:03.1", "40:03.1", "40:03.1", "40:03.2", "40:03.2", "40:03.2", "40:03.3", "40:03.3", "40:03.3", "40:03.4", "40:03.4", "40:03.4", "40:03.5", "40:03.5", "40:03.5", "40:03.6", "40:03.6", "40:03.6", "40:03.7", "40:03.7", "40:03.7", "40:03.8", "40:03.8", "40:03.8", "40:03.9", "40:03.9", "40:03.9", "40:04.0", "40:04.0", "40:04.0", "40:04.1", "40:04.1", "40:04.1", "40:04.2", "40:04.2", "40:04.2", "40:04.3", "40:04.3", "40:04.3", "40:04.4", "40:04.4", "40:04.4", "40:04.5", "40:04.5", "40:04.5", "40:04.6", "40:04.6", "40:04.6", "40:04.7", "40:04.7", "40:04.7", "40:04.8", "40:04.8", "40:04.8", "40:04.9", "40:04.9", "40:04.9", "40:05.0", "40:05.0", "40:05.0", "40:05.1", "40:05.1", "40:05.1", "40:05.2", "40:05.2", "40:05.2", "40:05.3", "40:05.3", "40:05.3", "40:05.4", "40:05.4", "40:05.4", "40:05.5", "40:05.5", "40:05.5", "40:05.6", "40:05.6", "40:05.6", "40:05.7", "40:05.7", "40:05.7", "40:05.8", "40:05.8", "40:05.8", "40:05.9", "40:05.9", "40:05.9", "40:06.0", "40:06.0", "40:06.0", "40:06.1", "40:06.1", "40:06.1", "40:06.2", "40:06.2", "40:06.2", "40:06.3", "40:06.3", "40:06.3", "40:06.4", "40:06.4", "40:06.4", "40:06.5", "40:06.5", "40:06.5", "40:06.6", "40:06.6", "40:06.6", "40:06.7", "40:06.7", "40:06.7", "40:06.8", "40:06.8", "40:06.8", "40:06.9", "40:06.9", "40:06.9", "40:07.0", "40:07.0", "40:07.0", "40:07.1", "40:07.1", "40:07.1", "40:07.2", "40:07.2", "40:07.2", "40:07.3", "40:07.3", "40:07.3", "40:07.4", "40:07.4", "40:07.4", "40:07.5", "40:07.5", "40:07.5", "40:07.6", "40:07.6", "40:07.6", "40:07.7", "40:07.7", "40:07.7", "40:07.8", "40:07.8", "40:07.8", "40:07.9", "40:07.9", "40:07.9", "40:08.0", "40:08.0", "40:08.0", "40:08.1", "40:08.1", "40:08.1", "40:08.2", "40:08.2", "40:08.2", "40:08.3", "40:08.3", "40:08.3", "40:08.4", "40:08.4", "40:08.4", "40:08.5", "40:08.5", "40:08.5", "40:08.6", "40:08.6", "40:08.6", "40:08.7", "40:08.7", "40:08.7", "40:08.8", "40:08.8", "40:08.8", "40:08.9", "40:08.9", "40:08.9", "40:09.0", "40:09.0", "40:09.0", "40:09.1", "40:09.1", "40:09.1", "40:09.2", "40:09.2", "40:09.2", "40:09.3", "40:09.3", "40:09.3", "40:09.4", "40:09.4", "40:09.4", "40:09.5", "40:09.5", "40:09.5", "40:09.6", "40:09.6", "40:09.6", "40:09.7", "40:09.7", "40:09.7", "40:09.8", "40:09.8", "40:09.8", "40:09.9", "40:09.9", "40:09.9", "40:10.0", "40:10.0", "40:10.0", "40:10.1", "40:10.1", "40:10.1", "40:10.2", "40:10.2", "40:10.2", "40:10.3", "40:10.3", "40:10.3", "40:10.4", "40:10.4", "40:10.4", "40:10.5", "40:10.5", "40:10.5", "40:10.6", "40:10.6", "40:10.6", "40:10.7", "40:10.7", "40:10.7", "40:10.8", "40:10.8", "40:10.8", "40:10.9", "40:10.9", "40:10.9", "40:11.0", "40:11.0", "40:11.0", "40:11.1", "40:11.1", "40:11.1", "40:11.2", "40:11.2", "40:11.2", "40:11.3", "40:11.3", "40:11.3", "40:11.4", "40:11.4", "40:11.4", "40:11.5", "40:11.5", "40:11.5", "40:11.6", "40:11.6", "40:11.6", "40:11.7", "40:11.7", "40:11.7", "40:11.8", "40:11.8", "40:11.8", "40:11.9", "40:11.9", "40:11.9", "40:12.0", "40:12.0", "40:12.0", "40:12.1", "40:12.1", "40:12.1", "40:12.2", "40:12.2", "40:12.2", "40:12.3", "40:12.3", "40:12.3", "40:12.4", "40:12.4", "40:12.4", "40:12.5", "40:12.5", "40:12.5", "40:12.6", "40:12.6", "40:12.6", "40:12.7", "40:12.7", "40:12.7", "40:12.8", "40:12.8", "40:12.8", "40:12.9", "40:12.9", "40:12.9", "40:13.0", "40:13.0", "40:13.0", "40:13.1", "40:13.1", "40:13.1", "40:13.2", "40:13.2", "40:13.2", "40:13.3", "40:13.3", "40:13.3", "40:13.4", "40:13.4", "40:13.4", "40:13.5", "40:13.5", "40:13.5", "40:13.6", "40:13.6", "40:13.6", "40:13.7", "40:13.7", "40:13.7", "40:13.8", "40:13.8", "40:13.8", "40:13.9", "40:13.9", "40:13.9", "40:14.0", "40:14.0", "40:14.0", "40:14.1", "40:14.1", "40:14.1", "40:14.2", "40:14.2", "40:14.2", "40:14.3", "40:14.3", "40:14.3", "40:14.4", "40:14.4", "40:14.4", "40:14.5", "40:14.5", "40:14.5", "40:14.6", "40:14.6", "40:14.6", "40:14.7", "40:14.7", "40:14.7", "40:14.8", "40:14.8", "40:14.8", "40:14.9", "40:14.9", "40:14.9", "40:15.0", "40:15.0", "40:15.0", "40:15.1", "40:15.1", "40:15.1", "40:15.2", "40:15.2", "40:15.2", "40:15.3", "40:15.3", "40:15.3", "40:15.4", "40:15.4", "40:15.4", "40:15.5", "40:15.5", "40:15.5", "40:15.6", "40:15.6", "40:15.6", "40:15.7", "40:15.7", "40:15.7", "40:15.8", "40:15.8", "40:15.8", "40:15.9", "40:15.9", "40:15.9", "40:16.0", "40:16.0", "40:16.0", "40:16.1", "40:16.1", "40:16.1", "40:16.2", "40:16.2", "40:16.2", "40:16.3", "40:16.3", "40:16.3", "40:16.4", "40:16.4", "40:16.4", "40:16.5", "40:16.5", "40:16.5", "40:16.6", "40:16.6", "40:16.6", "40:16.7", "40:16.7", "40:16.7", "40:16.8", "40:16.8", "40:16.8", "40:16.9", "40:16.9", "40:16.9", "40:17.0", "40:17.0", "40:17.0", "40:17.1", "40:17.1", "40:17.1", "40:17.2", "40:17.2", "40:17.2", "40:17.3", "40:17.3", "40:17.3", "40:17.4", "40:17.4", "40:17.4", "40:17.5", "40:17.5", "40:17.5", "40:17.6", "40:17.6", "40:17.6", "40:17.7", "40:17.7", "40:17.7", "40:17.8", "40:17.8", "40:17.8", "40:17.9", "40:17.9", "40:17.9", "40:18.0", "40:18.0", "40:18.0", "40:18.1", "40:18.1", "40:18.1", "40:18.2", "40:18.2", "40:18.2", "40:18.3", "40:18.3", "40:18.3", "40:18.4", "40:18.4", "40:18.4", "40:18.5", "40:18.5", "40:18.5", "40:18.6", "40:18.6", "40:18.6", "40:18.7", "40:18.7", "40:18.7", "40:18.8", "40:18.8", "40:18.8", "40:18.9", "40:18.9", "40:18.9", "40:19.0", "40:19.0", "40:19.0", "40:19.1", "40:19.1", "40:19.1", "40:19.2", "40:19.2", "40:19.2", "40:19.3", "40:19.3", "40:19.3", "40:19.4", "40:19.4", "40:19.4", "40:19.5", "40:19.5", "40:19.5", "40:19.6", "40:19.6", "40:19.6", "40:19.7", "40:19.7", "40:19.7", "40:19.8", "40:19.8", "40:19.8", "40:19.9", "40:19.9", "40:19.9", "40:20.0", "40:20.0", "40:20.0", "40:20.1", "40:20.1", "40:20.1", "40:20.2", "40:20.2", "40:20.2", "40:20.3", "40:20.3", "40:20.3", "40:20.4", "40:20.4", "40:20.4", "40:20.5", "40:20.5", "40:20.5", "40:20.6", "40:20.6", "40:20.6", "40:20.7", "40:20.7", "40:20.7", "40:20.8", "40:20.8", "40:20.8", "40:20.9", "40:20.9", "40:20.9", "40:21.0", "40:21.0", "40:21.0", "40:21.1", "40:21.1", "40:21.1", "40:21.2", "40:21.2", "40:21.2", "40:21.3", "40:21.3", "40:21.3", "40:21.4", "40:21.4", "40:21.4", "40:21.5", "40:21.5", "40:21.5", "40:21.6", "40:21.6", "40:21.6", "40:21.7", "40:21.7", "40:21.7", "40:21.8", "40:21.8", "40:21.8", "40:21.9", "40:21.9", "40:21.9", "40:22.0", "40:22.0", "40:22.0", "40:22.1", "40:22.1", "40:22.1", "40:22.2", "40:22.2", "40:22.2", "40:22.3", "40:22.3", "40:22.3", "40:22.4", "40:22.4", "40:22.4", "40:22.5", "40:22.5", "40:22.5", "40:22.6", "40:22.6", "40:22.6", "40:22.7", "40:22.7", "40:22.7", "40:22.8", "40:22.8", "40:22.8", "40:22.9", "40:22.9", "40:22.9", "40:23.0", "40:23.0", "40:23.0", "40:23.1", "40:23.1", "40:23.1", "40:23.2", "40:23.2", "40:23.2", "40:23.3", "40:23.3", "40:23.3", "40:23.4", "40:23.4", "40:23.4", "40:23.5", "40:23.5", "40:23.5", "40:23.6", "40:23.6", "40:23.6", "40:23.7", "40:23.7", "40:23.7", "40:23.8", "40:23.8", "40:23.8", "40:23.9", "40:23.9", "40:23.9", "40:24.0", "40:24.0", "40:24.0", "40:24.1", "40:24.1", "40:24.1", "40:24.2", "40:24.2", "40:24.2", "40:24.3", "40:24.3", "40:24.3", "40:24.4", "40:24.4", "40:24.4", "40:24.5", "40:24.5", "40:24.5", "40:24.6", "40:24.6", "40:24.6", "40:24.7", "40:24.7", "40:24.7", "40:24.8", "40:24.8", "40:24.8", "40:24.9", "40:24.9", "40:24.9", "40:25.0", "40:25.0", "40:25.0", "40:25.1", "40:25.1", "40:25.1", "40:25.2", "40:25.2", "40:25.2", "40:25.3", "40:25.3", "40:25.3", "40:25.4", "40:25.4", "40:25.4", "40:25.5", "40:25.5", "40:25.5", "40:25.6", "40:25.6", "40:25.6", "40:25.7", "40:25.7", "40:25.7", "40:25.8", "40:25.8", "40:25.8", "40:25.9", "40:25.9", "40:25.9", "40:26.0", "40:26.0", "40:26.0", "40:26.1", "40:26.1", "40:26.1", "40:26.2", "40:26.2", "40:26.2", "40:26.3", "40:26.3", "40:26.3", "40:26.4", "40:26.4", "40:26.4", "40:26.5", "40:26.5", "40:26.5", "40:26.6", "40:26.6", "40:26.6", "40:26.7", "40:26.7", "40:26.7", "40:26.8", "40:26.8", "40:26.8", "40:26.9", "40:26.9", "40:26.9", "40:27.0", "40:27.0", "40:27.0", "40:27.1", "40:27.1", "40:27.1", "40:27.2", "40:27.2", "40:27.2", "40:27.3", "40:27.3", "40:27.3", "40:27.4", "40:27.4", "40:27.4", "40:27.5", "40:27.5", "40:27.5", "40:27.6", "40:27.6", "40:27.6", "40:27.7", "40:27.7", "40:27.7", "40:27.8", "40:27.8", "40:27.8", "40:27.9", "40:27.9", "40:27.9", "40:28.0", "40:28.0", "40:28.0", "40:28.1", "40:28.1", "40:28.1", "40:28.2", "40:28.2", "40:28.2", "40:28.3", "40:28.3", "40:28.3", "40:28.4", "40:28.4", "40:28.4", "40:28.5", "40:28.5", "40:28.5", "40:28.6", "40:28.6", "40:28.6", "40:28.7", "40:28.7", "40:28.7", "40:28.8", "40:28.8", "40:28.8", "40:28.9", "40:28.9", "40:28.9", "40:29.0", "40:29.0", "40:29.0", "40:29.1", "40:29.1", "40:29.1", "40:29.2", "40:29.2", "40:29.2", "40:29.3", "40:29.3", "40:29.3", "40:29.4", "40:29.4", "40:29.4", "40:29.5", "40:29.5", "40:29.5", "40:29.6", "40:29.6", "40:29.6", "40:29.7", "40:29.7", "40:29.7", "40:29.8", "40:29.8", "40:29.8", "40:29.9", "40:29.9", "40:29.9", "40:30.0", "40:30.0", "40:30.0", "40:30.1", "40:30.1", "40:30.1", "40:30.2", "40:30.2", "40:30.2", "40:30.3", "40:30.3", "40:30.3", "40:30.4", "40:30.4", "40:30.4", "40:30.5", "40:30.5", "40:30.5", "40:30.6", "40:30.6", "40:30.6", "40:30.7", "40:30.7", "40:30.7", "40:30.8", "40:30.8", "40:30.8", "40:30.9", "40:30.9", "40:30.9", "40:31.0", "40:31.0", "40:31.0", "40:31.1", "40:31.1", "40:31.1", "40:31.2", "40:31.2", "40:31.2", "40:31.3", "40:31.3", "40:31.3", "40:31.4", "40:31.4", "40:31.4", "40:31.5", "40:31.5", "40:31.5", "40:31.6", "40:31.6", "40:31.6", "40:31.7", "40:31.7", "40:31.7", "40:31.8", "40:31.8", "40:31.8", "40:31.9", "40:31.9", "40:31.9", "40:32.0", "40:32.0", "40:32.0", "40:32.1", "40:32.1", "40:32.1", "40:32.2", "40:32.2", "40:32.2", "40:32.3", "40:32.3", "40:32.3", "40:32.4", "40:32.4", "40:32.4", "40:32.5", "40:32.5", "40:32.5", "40:32.6", "40:32.6", "40:32.6", "40:32.7", "40:32.7", "40:32.7", "40:32.8", "40:32.8", "40:32.8", "40:32.9", "40:32.9", "40:32.9", "40:33.0", "40:33.0", "40:33.0", "40:33.1", "40:33.1", "40:33.1", "40:33.2", "40:33.2", "40:33.2", "40:33.3", "40:33.3", "40:33.3", "40:33.4", "40:33.4", "40:33.4", "40:33.5", "40:33.5", "40:33.5", "40:33.6", "40:33.6", "40:33.6", "40:33.7", "40:33.7", "40:33.7", "40:33.8", "40:33.8", "40:33.8", "40:33.9", "40:33.9", "40:33.9", "40:34.0", "40:34.0", "40:34.0", "40:34.1", "40:34.1", "40:34.1", "40:34.2", "40:34.2", "40:34.2", "40:34.3", "40:34.3", "40:34.3", "40:34.4", "40:34.4", "40:34.4", "40:34.5", "40:34.5", "40:34.5", "40:34.6", "40:34.6", "40:34.6", "40:34.7", "40:34.7", "40:34.7", "40:34.8", "40:34.8", "40:34.8", "40:34.9", "40:34.9", "40:34.9", "40:35.0", "40:35.0", "40:35.0", "40:35.1", "40:35.1", "40:35.1", "40:35.2", "40:35.2", "40:35.2", "40:35.3", "40:35.3", "40:35.3", "40:35.4", "40:35.4", "40:35.4", "40:35.5", "40:35.5", "40:35.5", "40:35.6", "40:35.6", "40:35.6", "40:35.7", "40:35.7", "40:35.7", "40:35.8", "40:35.8", "40:35.8", "40:35.9", "40:35.9", "40:35.9", "40:36.0", "40:36.0", "40:36.0", "40:36.1", "40:36.1", "40:36.1", "40:36.2", "40:36.2", "40:36.2", "40:36.3", "40:36.3", "40:36.3", "40:36.4", "40:36.4", "40:36.4", "40:36.5", "40:36.5", "40:36.5", "40:36.6", "40:36.6", "40:36.6", "40:36.7", "40:36.7", "40:36.7", "40:36.8", "40:36.8", "40:36.8", "40:36.9", "40:36.9", "40:36.9", "40:37.0", "40:37.0", "40:37.0", "40:37.1", "40:37.1", "40:37.1", "40:37.2", "40:37.2", "40:37.2", "40:37.3", "40:37.3", "40:37.3", "40:37.4", "40:37.4", "40:37.4", "40:37.5", "40:37.5", "40:37.5", "40:37.6", "40:37.6", "40:37.6", "40:37.7", "40:37.7", "40:37.7", "40:37.8", "40:37.8", "40:37.8", "40:37.9", "40:37.9", "40:37.9", "40:38.0", "40:38.0", "40:38.0", "40:38.1", "40:38.1", "40:38.1", "40:38.2", "40:38.2", "40:38.2", "40:38.3", "40:38.3", "40:38.3", "40:38.4", "40:38.4", "40:38.4", "40:38.5", "40:38.5", "40:38.5", "40:38.6", "40:38.6", "40:38.6", "40:38.7", "40:38.7", "40:38.7", "40:38.8", "40:38.8", "40:38.8", "40:38.9", "40:38.9", "40:38.9", "40:39.0", "40:39.0", "40:39.0", "40:39.1", "40:39.1", "40:39.1", "40:39.2", "40:39.2", "40:39.2", "40:39.3", "40:39.3", "40:39.3", "40:39.4", "40:39.4", "40:39.4", "40:39.5", "40:39.5", "40:39.5", "40:39.6", "40:39.6", "40:39.6", "40:39.7", "40:39.7", "40:39.7", "40:39.8", "40:39.8", "40:39.8", "40:39.9", "40:39.9", "40:39.9", "40:40.0", "40:40.0", "40:40.0", "40:40.1", "40:40.1", "40:40.1", "40:40.2", "40:40.2", "40:40.2", "40:40.3", "40:40.3", "40:40.3", "40:40.4", "40:40.4", "40:40.4", "40:40.5", "40:40.5", "40:40.5", "40:40.6", "40:40.6", "40:40.6", "40:40.7", "40:40.7", "40:40.7", "40:40.8", "40:40.8", "40:40.8", "40:40.9", "40:40.9", "40:40.9", "40:41.0", "40:41.0", "40:41.0", "40:41.1", "40:41.1", "40:41.1", "40:41.2", "40:41.2", "40:41.2", "40:41.3", "40:41.3", "40:41.3", "40:41.4", "40:41.4", "40:41.4", "40:41.5", "40:41.5", "40:41.5", "40:41.6", "40:41.6", "40:41.6", "40:41.7", "40:41.7", "40:41.7", "40:41.8", "40:41.8", "40:41.8", "40:41.9", "40:41.9", "40:41.9", "40:42.0", "40:42.0", "40:42.0", "40:42.1", "40:42.1", "40:42.1", "40:42.2", "40:42.2", "40:42.2", "40:42.3", "40:42.3", "40:42.3", "40:42.4", "40:42.4", "40:42.4", "40:42.5", "40:42.5", "40:42.5", "40:42.6", "40:42.6", "40:42.6", "40:42.7", "40:42.7", "40:42.7", "40:42.8", "40:42.8", "40:42.8", "40:42.9", "40:42.9", "40:42.9", "40:43.0", "40:43.0", "40:43.0", "40:43.1", "40:43.1", "40:43.1", "40:43.2", "40:43.2", "40:43.2", "40:43.3", "40:43.3", "40:43.3", "40:43.4", "40:43.4", "40:43.4", "40:43.5", "40:43.5", "40:43.5", "40:43.6", "40:43.6", "40:43.6", "40:43.7", "40:43.7", "40:43.7", "40:43.8", "40:43.8", "40:43.8", "40:43.9", "40:43.9", "40:43.9", "40:44.0", "40:44.0", "40:44.0", "40:44.1", "40:44.1", "40:44.1", "40:44.2", "40:44.2", "40:44.2", "40:44.3", "40:44.3", "40:44.3", "40:44.4", "40:44.4", "40:44.4", "40:44.5", "40:44.5", "40:44.5", "40:44.6", "40:44.6", "40:44.6", "40:44.7", "40:44.7", "40:44.7", "40:44.8", "40:44.8", "40:44.8", "40:44.9", "40:44.9", "40:44.9", "40:45.0", "40:45.0", "40:45.0", "40:45.1", "40:45.1", "40:45.1", "40:45.2", "40:45.2", "40:45.2", "40:45.3", "40:45.3", "40:45.3", "40:45.4", "40:45.4", "40:45.4", "40:45.5", "40:45.5", "40:45.5", "40:45.6", "40:45.6", "40:45.6", "40:45.7", "40:45.7", "40:45.7", "40:45.8", "40:45.8", "40:45.8", "40:45.9", "40:45.9", "40:45.9", "40:46.0", "40:46.0", "40:46.0", "40:46.1", "40:46.1", "40:46.1", "40:46.2", "40:46.2", "40:46.2", "40:46.3", "40:46.3", "40:46.3", "40:46.4", "40:46.4", "40:46.4", "40:46.5", "40:46.5", "40:46.5", "40:46.6", "40:46.6", "40:46.6", "40:46.7", "40:46.7", "40:46.7", "40:46.8", "40:46.8", "40:46.8", "40:46.9", "40:46.9", "40:46.9", "40:47.0", "40:47.0", 
